vi "test_csm_helper.vi"() -> ()   [LabVIEW 2020]
uses:
  Typedef/Def-Argument Info.ctl
  <userlib>/_NEVSTOP/Communicable State Machine(CSM)/_Support/Priority Queue/Priority Queue.lvclass/Priority Queue.ctl
  <userlib>/_NEVSTOP/Communicable State Machine(CSM)/Utility/Build Error Cluster.vi
  <userlib>/_NEVSTOP/Communicable State Machine(CSM)/_Support/Process/CSMP-Sync Call.vi
  <userlib>/_NEVSTOP/Communicable State Machine(CSM)/Utility/uuid.vi
  <userlib>/_NEVSTOP/Communicable State Machine(CSM)/Utility/Trim Both Whitespace.vi
  <userlib>/_NEVSTOP/Communicable State Machine(CSM)/_Support/Process/CSMP-Async Call.vi
  <userlib>/_NEVSTOP/Communicable State Machine(CSM)/_Support/GlobalEvent/GEvt-Generate Status Log.vi
  <userlib>/_NEVSTOP/Communicable State Machine(CSM)/_Support/Process/CSMP-Broadcast.vi
  <userlib>/_NEVSTOP/Communicable State Machine(CSM)/_Support/GlobalEvent/GEvt-Generate Interrupt Log.vi
  <userlib>/_NEVSTOP/Communicable State Machine(CSM)/_Support/GlobalEvent/GEvt-Generate Register Log.vi
  <userlib>/_NEVSTOP/Communicable State Machine(CSM)/_Support/Process/CSMP-Register Status.vi
  <userlib>/_NEVSTOP/Communicable State Machine(CSM)/_Support/GlobalEvent/GEvt-Generate Unregister Log.vi
  <userlib>/_NEVSTOP/Communicable State Machine(CSM)/_Support/Process/CSMP-Unregister Status.vi
  <userlib>/_NEVSTOP/Communicable State Machine(CSM)/_Support/CSMQ/_CSMObj-Unlock.vi
  <userlib>/_NEVSTOP/Communicable State Machine(CSM)/_Support/Process/CSMP-PostPostMsg.vi
  <userlib>/_NEVSTOP/Communicable State Machine(CSM)/_Support/Process/CSMP-PostSendMsg.vi
  <userlib>/_NEVSTOP/Communicable State Machine(CSM)/_Support/CSMQ/_CSMObj-Lock State.vi
  <userlib>/_NEVSTOP/Communicable State Machine(CSM)/_Support/Common/Splite Reason String Part.vi
  <userlib>/_NEVSTOP/Communicable State Machine(CSM)/_Support/Common/Trim Single line Text.vi
  <userlib>/_NEVSTOP/Communicable State Machine(CSM)/_Support/CSMQ/_CSMOFGV Release.vi
  <userlib>/_NEVSTOP/Communicable State Machine(CSM)/_Support/Common/Remove Comments from Line.vi
  <userlib>/_NEVSTOP/Communicable State Machine(CSM)/_Support/Common/Splite Single-line Message.vi
  <userlib>/_NEVSTOP/Communicable State Machine(CSM)/_Support/Common/Parse Next Single-line State.vi
  <userlib>/_NEVSTOP/Communicable State Machine(CSM)/_Support/CSMQ/_CSMOFGV Dequeue.vi
  <userlib>/_NEVSTOP/Communicable State Machine(CSM)/_Support/CSMQ/_CSMObj-Log Error if in a Remote Session.vi
  <userlib>/_NEVSTOP/Communicable State Machine(CSM)/_Support/GlobalEvent/GEvt-Generate State Change Log.vi
  <userlib>/_NEVSTOP/Communicable State Machine(CSM)/_Support/GlobalEvent/GEvt-Generate Remaining States Log.vi
  <userlib>/_NEVSTOP/Communicable State Machine(CSM)/_Support/GlobalEvent/GEvt-Generate Module Destroyed Log.vi
  <userlib>/_NEVSTOP/Communicable State Machine(CSM)/_Support/GlobalEvent/GEvt-Generate Complete Log.vi
  <userlib>/_NEVSTOP/Communicable State Machine(CSM)/_Support/GlobalEvent/GEvt-Generate Module Created Log.vi
  <userlib>/_NEVSTOP/Communicable State Machine(CSM)/AdvanceAPI/CSM - Revert Arguments-Safe String.vi
  <userlib>/_NEVSTOP/Communicable State Machine(CSM)/AdvanceAPI/CSM - Make String Arguments Safe.vi
  <userlib>/_NEVSTOP/Communicable State Machine(CSM)/_Support/CSMQ/_CSMObj-Message Check.vi
  <userlib>/_NEVSTOP/Communicable State Machine(CSM)/_Support/CSMQ/_CSMObj-Enqueue Cross-Module Message.vi
  <userlib>/_NEVSTOP/Communicable State Machine(CSM)/_Support/CSMQ/_CSMOFGV Get.vi
  <userlib>/_NEVSTOP/Communicable State Machine(CSM)/_Support/FGV-BroadcastRegistry/Cache-Broadcast Registry Search Result.vi
  <userlib>/_NEVSTOP/Communicable State Machine(CSM)/AdvanceAPI/CSM - Register Status Change.vi
  <userlib>/_NEVSTOP/Communicable State Machine(CSM)/AdvanceAPI/CSM - Unregister Status Change.vi
  <userlib>/_NEVSTOP/Communicable State Machine(CSM)/_Support/Common/Hex Str to U8 Data.vi
  <userlib>/_NEVSTOP/Communicable State Machine(CSM)/_Support/Common/Concatenate State with Arguments.vi
  <userlib>/_NEVSTOP/Communicable State Machine(CSM)/_Support/Common/U8 Data to Hex Str.vi
  <userlib>/_NEVSTOP/Communicable State Machine(CSM)/_Support/Priority Queue/Dequeue Element.vi
  <userlib>/_NEVSTOP/Communicable State Machine(CSM)/AdvanceAPI/CSM - Keywords.vi
  <userlib>/_NEVSTOP/Communicable State Machine(CSM)/_Support/Priority Queue/Enqueue Element.vi
  <userlib>/_NEVSTOP/Communicable State Machine(CSM)/_Support/GlobalEvent/FGV-GlobalEventRef.vi
  <userlib>/_NEVSTOP/Communicable State Machine(CSM)/_Support/CSMQ/_CSMOFGV Obtain.vi
  <userlib>/_NEVSTOP/Communicable State Machine(CSM)/_Support/CSMQ/_CSMOFGV.vi
  <userlib>/_NEVSTOP/Communicable State Machine(CSM)/_Support/GlobalEvent/FGV-StatusChangeEventRef.vi
  <userlib>/_NEVSTOP/Communicable State Machine(CSM)/_Support/FGV-BroadcastRegistry/global-CSMQ FGV Change Flag.vi
  <userlib>/_NEVSTOP/Communicable State Machine(CSM)/_Support/FGV-BroadcastRegistry/global-Broadcast Cache Change Flag.vi
  <userlib>/_NEVSTOP/Communicable State Machine(CSM)/_Support/BroadcastRegistry/HelperVI/Broadcast Item Key.vi
  <userlib>/_NEVSTOP/Communicable State Machine(CSM)/_Support/FGV-BroadcastRegistry/FGV-BroadcastRegistry.vi
  <userlib>/_NEVSTOP/Communicable State Machine(CSM)/_Support/Message/Parse Register Message.vi
  <userlib>/_NEVSTOP/Communicable State Machine(CSM)/_Support/Message/Parse Unregister Message.vi
  API/Create From VI Reference.vi
  <userlib>/_NEVSTOP/Communicable State Machine(CSM)/Communicable State Machine.lvlib
  CSM-Helper.lvclass
panel:
  out "Array 3":cluster{string, "Argument":T1, "Response":T1}[](array[cluster])
  out "Array 2":string[](array[string])
  out "Array":string[](array[string])
  out "State History":string
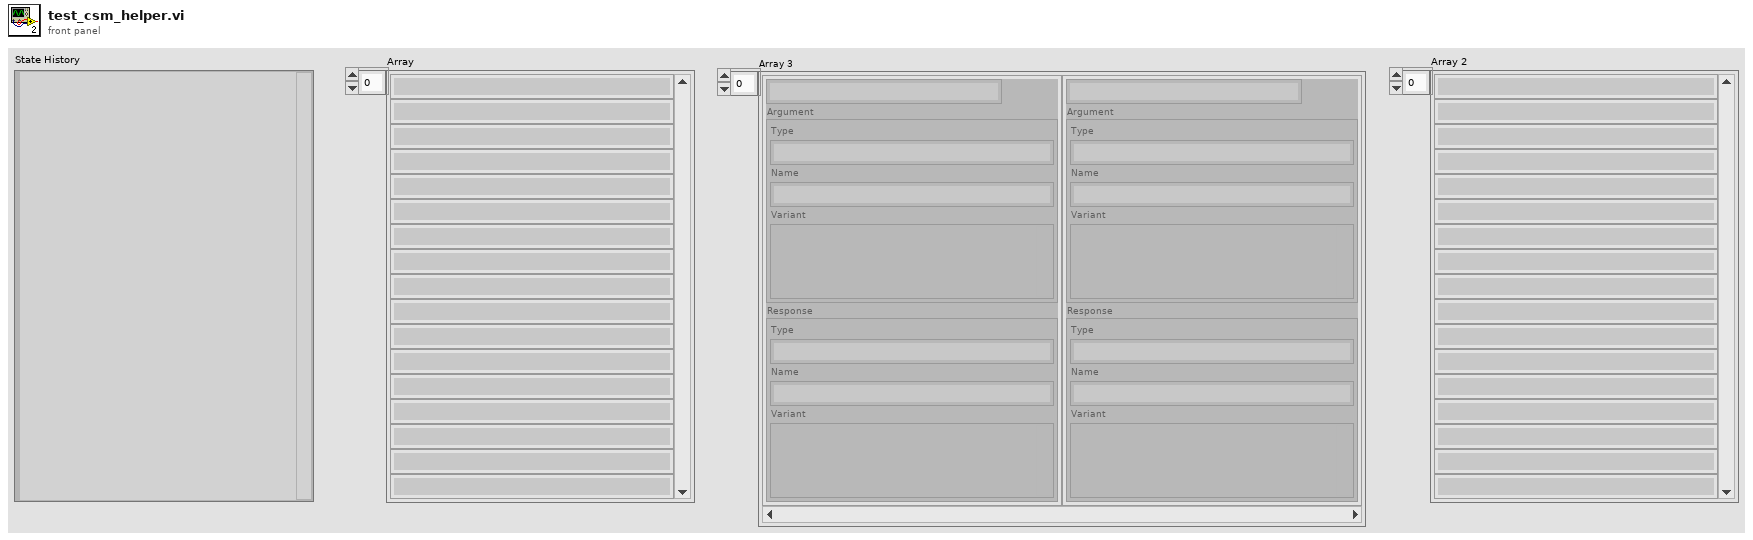
[diagram p1: front panel]
types:
  T1 = typedef "CSM-Helper.lvclass/Def-Argument Info.ctl" = cluster{"Type":string, "Name":string, "Variant":variant}
  T2 = enum32{"Invalid", "Standard", "Closed", "Hidden", "Minimized", "Maximized"}
  T3 = enum32{"invalid app kind", "Development System", "Run Time System", "Student Edition", "Embedded LabVIEW", "Evaluation", "Custom"}
  T4 = typedef "Communicable State Machine.lvlib/_CSM_Response Source Message.ctl" = cluster{"‘State":string, "’Arguments":string, "’Error":errorcluster}
  T5 = cluster{"Core":cluster{"Current VI Reference":refnum<vi>, "Close Panel on Exit?":bool}, "Your Boolean data":bool, "Your string data":string}
  T6 = cluster{"Current VI Reference":refnum<vi>, "Close Panel on Exit?":bool}
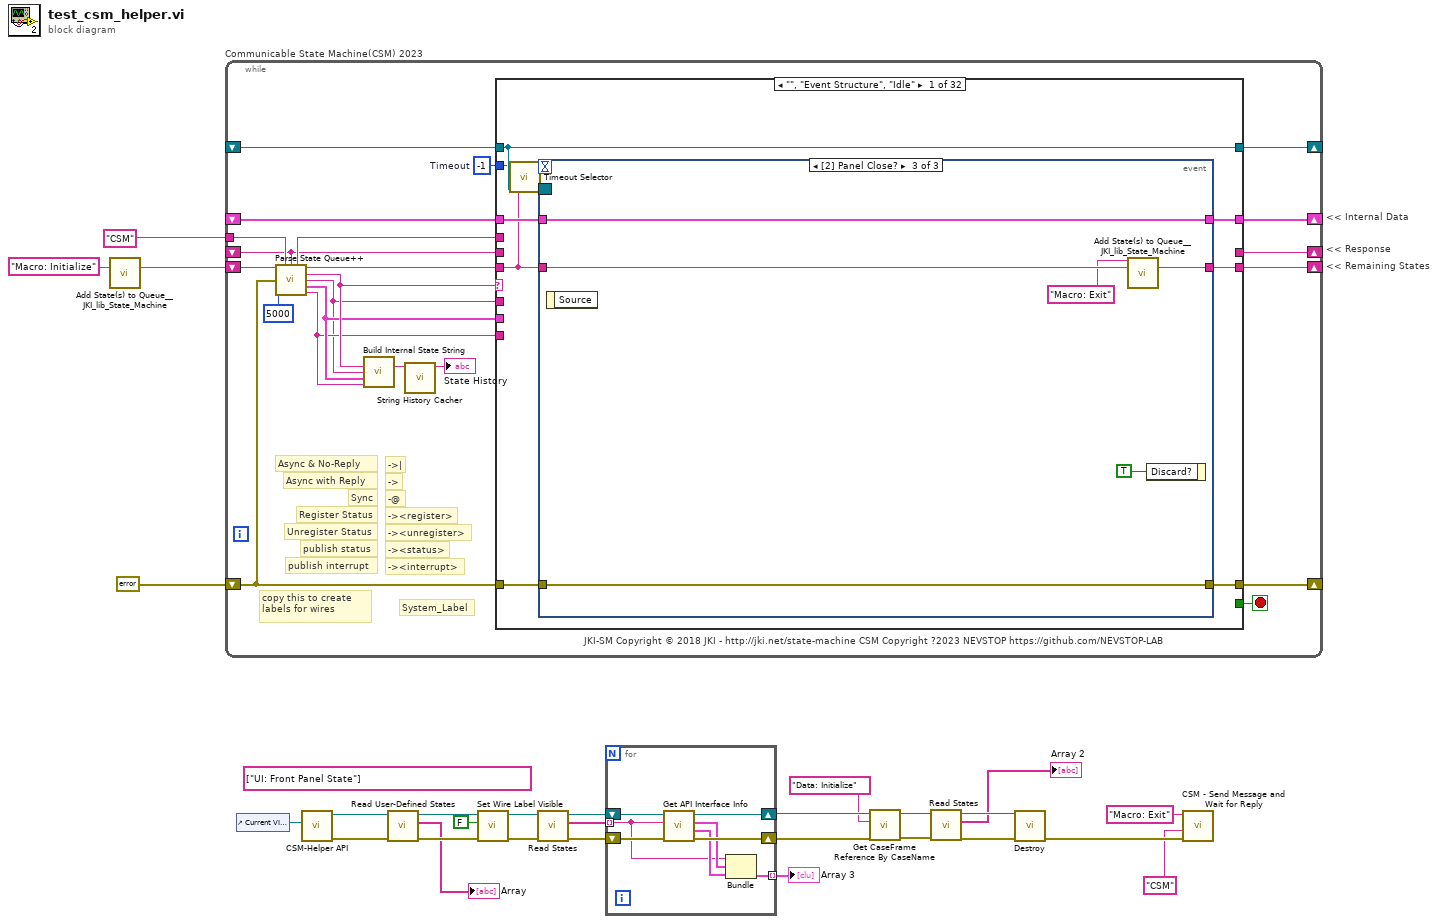
[diagram p0: block diagram]
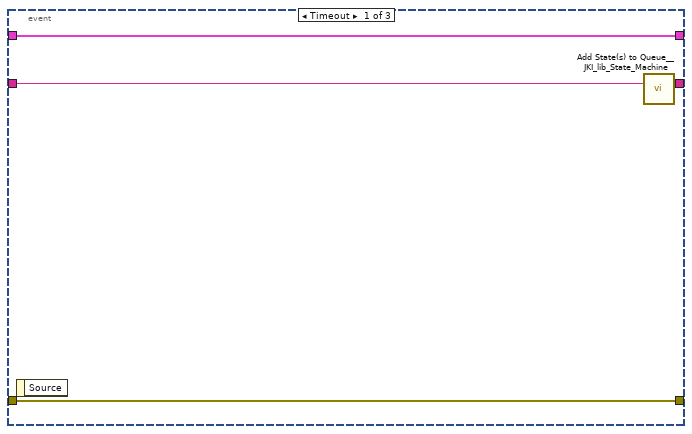
[diagram p2: hidden frame]
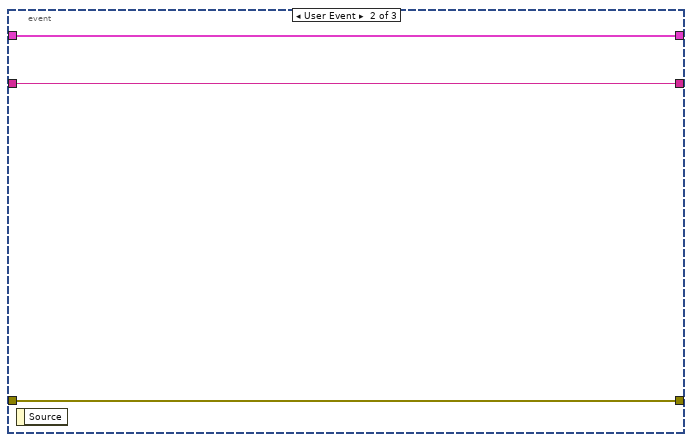
[diagram p3: hidden frame]
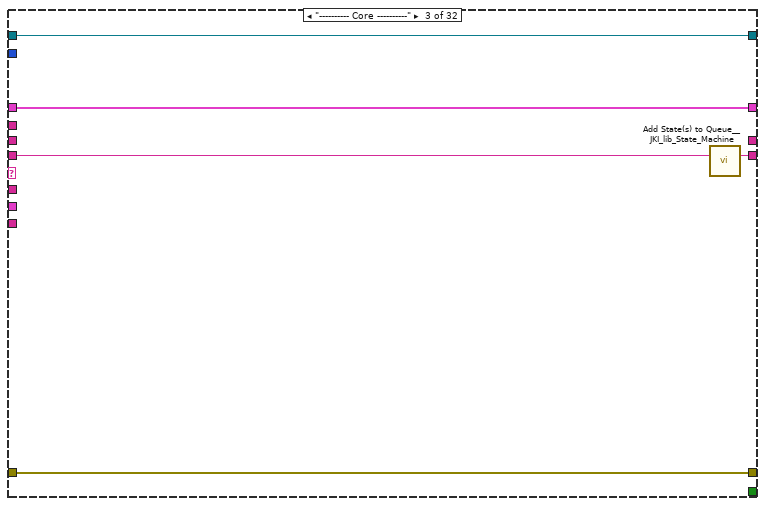
[diagram p5: hidden frame]
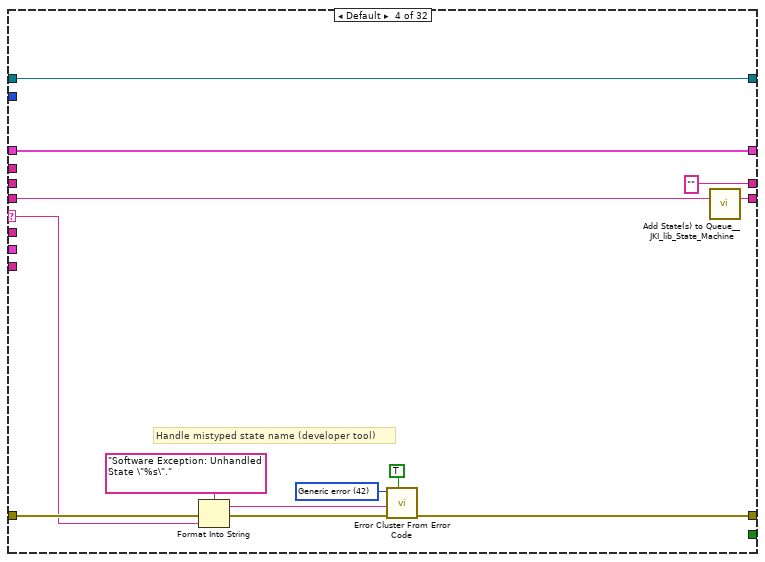
[diagram p6: hidden frame]
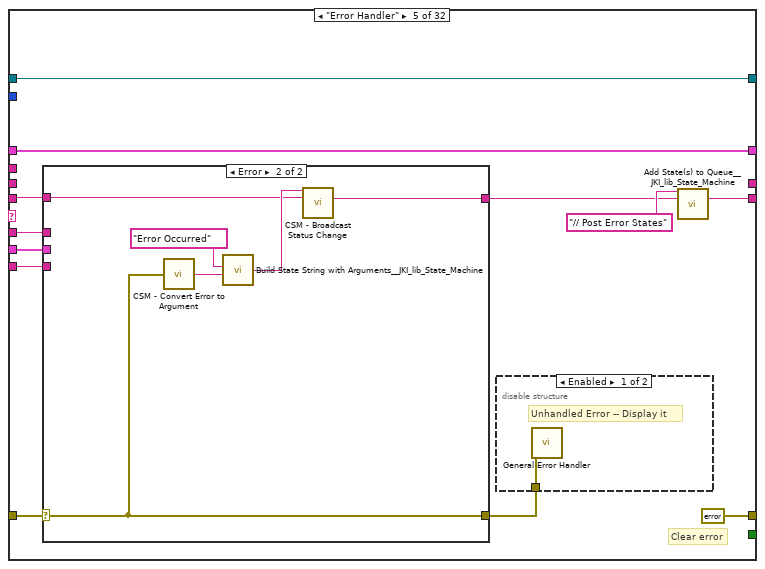
[diagram p7: hidden frame]
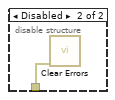
[diagram p8: hidden frame]
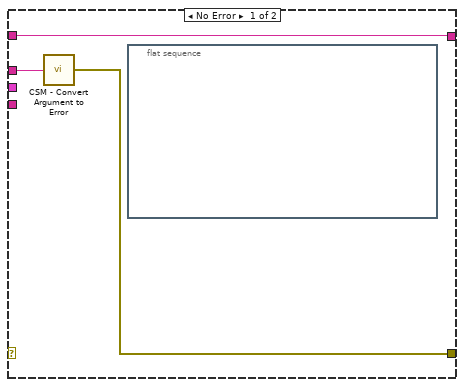
[diagram p9: hidden frame]
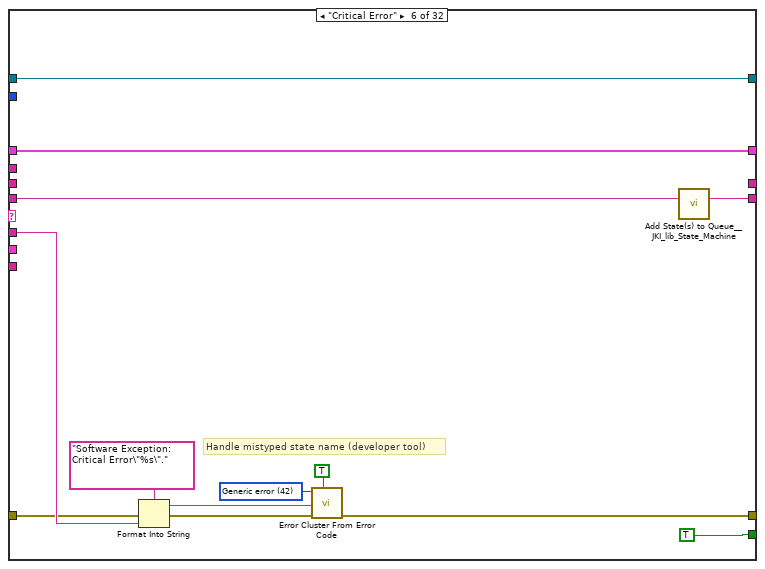
[diagram p10: hidden frame]
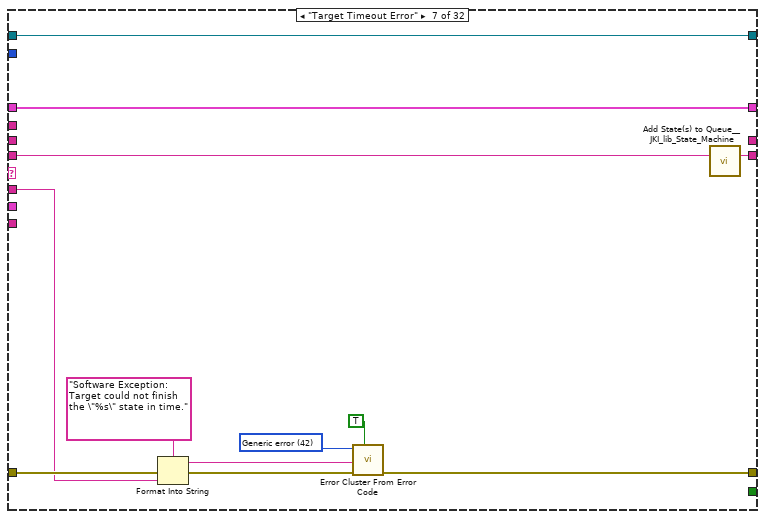
[diagram p11: hidden frame]
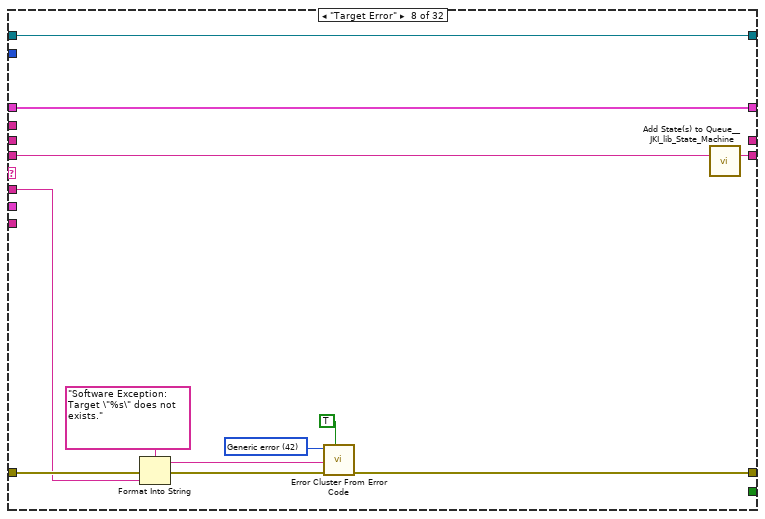
[diagram p12: hidden frame]
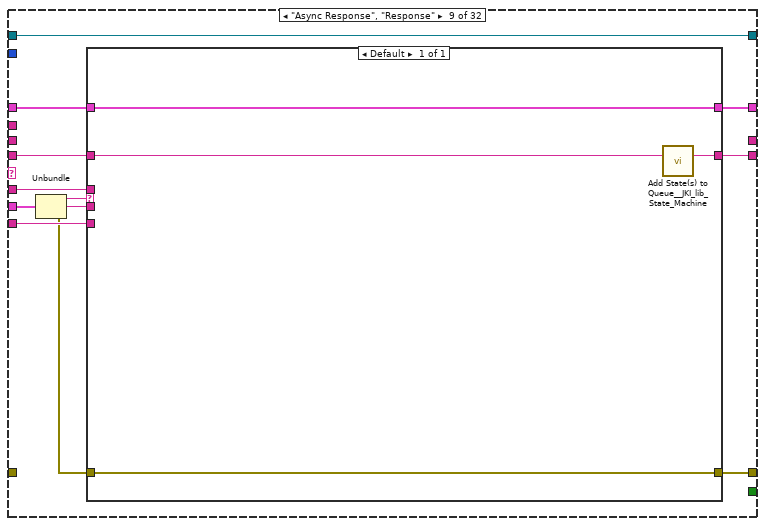
[diagram p13: hidden frame]
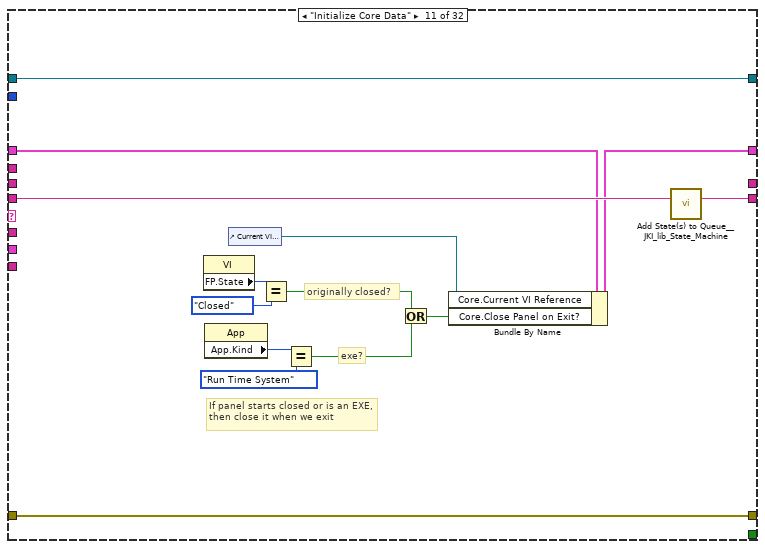
[diagram p15: hidden frame]
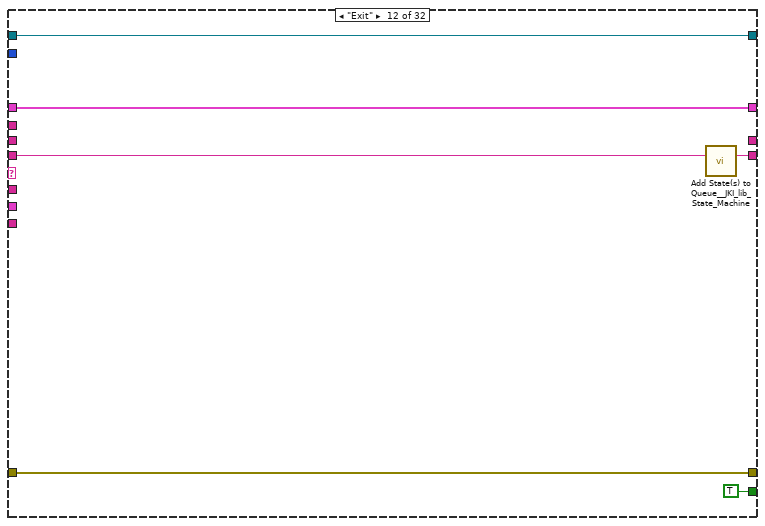
[diagram p16: hidden frame]
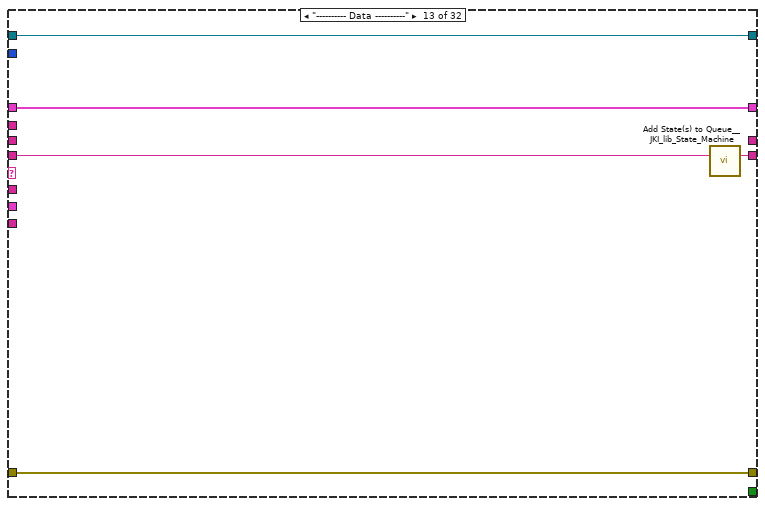
[diagram p17: hidden frame]
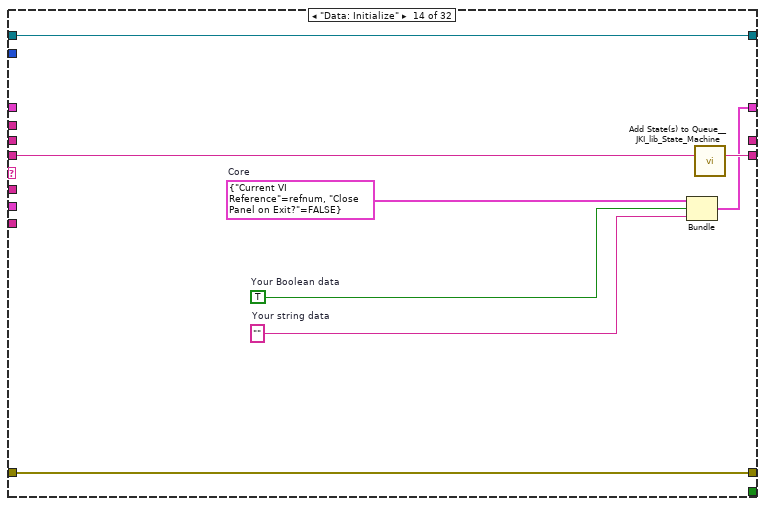
[diagram p18: hidden frame]
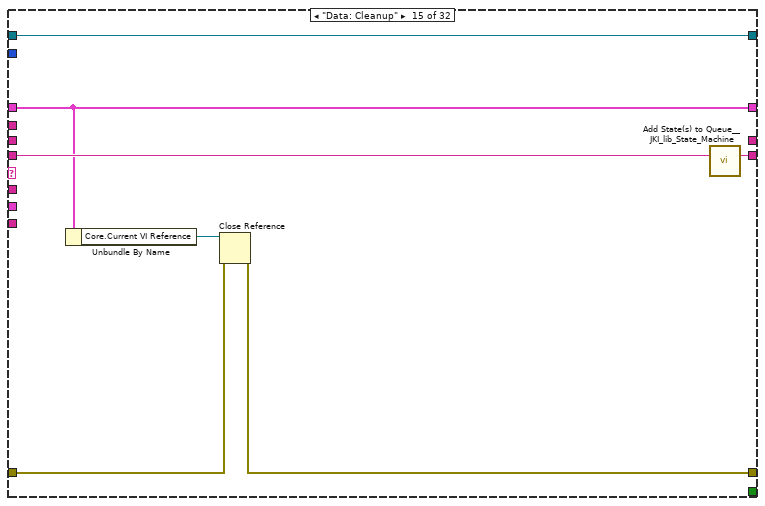
[diagram p19: hidden frame]
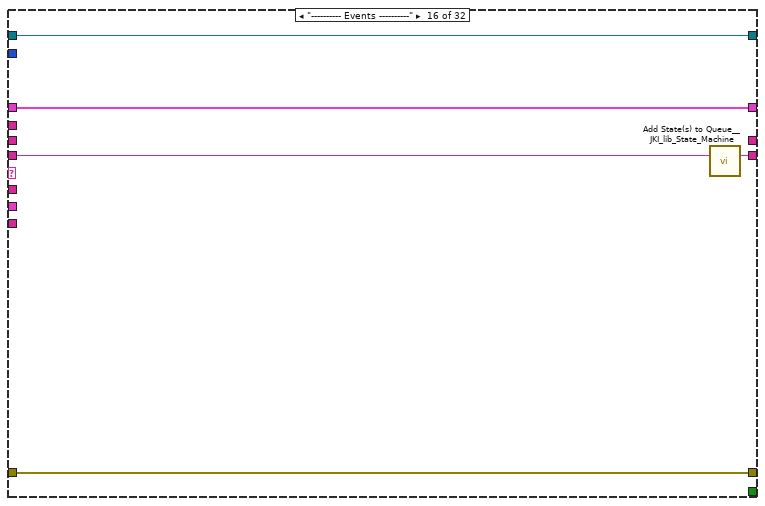
[diagram p20: hidden frame]
diagram:
  (unwired) string[] ["UI: Front Panel State"] ("Array")
  # "<< Internal Data"
  # "<< Response"
  # "<< Remaining States"
  n1 = call <vilib>:"Add State(s) to Queue__JKI_lib_State_Machine.vi"("State(s) in (\"\")"="Macro: Initialize" ("Init State(\"Macro: Initialize\")")) -> ("States Out"=w25:string)  [unwired: 14 in]
  n2 = while "Communicable State Machine(CSM) 2023" {
    shift-right: [w45] -> _
    shift-left: _ -> [w44]
    shift-right: [w48] -> _
    shift-left: errorcluster {"status"=FALSE, "code"=0, "source"=""} ("error out") -> [w42]
    shift-right: [w47] -> _
    shift-left: w25 -> [w49]
    tunnel: "CSM" ("Name(\"\" to use uuid)") -> [w37]
    shift-right: [w40] -> _
    shift-left: _ -> [w30]
    shift-right: [w39] -> _
    shift-left: _ -> [w38]
    stop <- w46 stop-if-true
    w43 = -1  # Timeout
    # "-><interrupt>"
    # "-><status>"
    # "-><unregister>"
    # "-><register>"
    # "-@"
    # "->"
    # "->|"
    # "publish interrupt"
    # "publish status"
    # "Unregister Status"
    # "Register Status"
    # "Sync"
    # "Async with Reply"
    # "Async & No-Reply"
    # "copy this to create labels for wires"
    # "System_Label"
    # "JKI-SM Copyright © 2018 JKI - http://jki.net/state-machine CSM Copyright ?2023 NEVSTOP https://github.com/NEVSTOP-LAB"
    n3 = call <userlib>:"Parse State Queue++.vi"("State Queue"=w49, "Name(\"\" to use uuid)"=w37, "Response Arguments"=w30, "Error In (no error)"=w42, "Response Timeout(5000ms)"=5000 ("Response Timeout(1000ms)")) -> ("Name Used"=w31:string, "Remaining States"=w50:string, "Current State"=w34:string, "Arguments"=w29:string, ">> Response Source Message >>"=w33:T4, ">> Source CSM >>"=w32:string)  [unwired: 5 in]
    n4 = call <userlib>:"Build Internal State String.vi"("State"=w34, "Arguments (\"\")"=w29, ">> Response Source Message >>"=w33, "Source (\"\")"=w32) -> ("State with Arguments"=w35:string)  [unwired: 11 in]
    n5 = call <userlib>:"String History Cacher.vi"("String"=w35) -> ("String Cache"=→"State History":string)  [unwired: 10 in]
    n6 = case shown="\"\", \"Event Structure\", \"Idle\"" w34 {
      selector: w34 -> [_ _ _ w84 _ _ _ _ _ _ _ _ _ _ _ _ _ _ _ _ _ _ _ _ _ _ _ _ _ _ _ _]
      tunnel: w50 -> [w51 w76 w81 w88 w99 w129 w137 w149 w164 w173 w188 w194 w199 w207 w214 w219 w226 w230 w236 w241 w248 w264 w334 w340 w352 w355 w361 w365 w369 w376 w381 w386]
      tunnel: w29 -> [_ _ _ _ w97 w122 w133 w145 w158 _ _ _ _ _ _ _ _ _ _ _ w243 w258 _ _ _ _ w357 _ _ _ _ _]
      tunnel: w44 -> [w58 w75 w78 w86 w105 w130 w135 w147 w162 w172 w181 w192 w196 _ w209 w216 w225 w229 w233 w239 w246 w260 w331 w337 w349 w354 w360 w364 w368 w373 w378 w383]
      tunnel: [w57 w74 w79 w90 errorcluster {"status"=FALSE, "code"=0, "source"=""} ("error out") w118 w131 w143 w161 w174 w185 w191 w197 w204 w210 w217 w220 w228 w234 w238 w244 w261 w332 w338 w350 w356 w362 w366 w370 w374 w379 w384] -> w48
      tunnel: w42 -> [w56 w74 w79 w89 w103 w119 w138 w150 _ w174 w185 w191 w197 w204 w211 w217 _ w231 w234 w238 w245 w262 w332 w338 w350 w356 w362 w366 w370 w374 w379 w384]
      tunnel: [w59 w76 w80 w87 w101 w128 w136 w148 w165 w173 w187 w193 w198 w206 w213 w218 w226 w230 w235 w240 w247 w263 w333 w339 w351 w355 w361 w365 w369 w375 w380 w385] -> w47
      tunnel: [_ _ _ _ _ TRUE _ _ _ _ _ TRUE _ _ _ _ _ _ _ _ _ _ _ _ _ _ _ _ _ _ _ _] -> w46
      tunnel: [w55 w75 w78 w86 w105 w130 w135 w147 w163 w172 w186 w192 w196 w205 w209 w216 w225 w229 w233 w239 w246 w260 w331 w337 w349 w354 w360 w364 w368 w373 w378 w383] -> w45
      tunnel: w43 -> [w53 _ _ _ _ _ _ _ _ _ _ _ _ _ _ _ _ _ _ _ _ _ _ _ _ _ _ _ _ _ _ _]
      tunnel: w32 -> [_ _ _ _ w96 _ _ _ w159 _ _ _ _ _ _ _ _ _ _ _ _ _ _ _ _ _ _ _ _ _ _ _]
      tunnel: w33 -> [_ _ _ _ w95 _ _ _ w160 _ _ _ _ _ _ _ _ _ _ _ _ _ _ _ _ _ _ _ _ _ _ _]
      tunnel: [_ _ _ "" _ _ _ _ _ _ _ _ _ _ _ _ _ _ _ _ _ _ _ _ _ _ "API1 Response" _ _ _ _ _] -> w40
      tunnel: [w54 w73 w77 w82 w104 w120 w132 w144 w166 w171 w175 w189 w195 w200 w208 w215 w224 w227 w232 w237 w242 w257 w330 w335 w342 w353 w359 w363 w367 w372 w377 w382] -> w39
      tunnel: w38 -> [w54 w73 w77 w82 w104 w120 w132 w144 w166 w171 w175 w189 w195 w200 w208 w215 _ w227 w232 w237 w242 w257 w330 w335 w342 w353 w359 w363 w367 w372 w377 w382]
      tunnel: w31 -> [_ _ _ _ _ _ _ _ _ _ _ _ _ _ _ _ w223 _ _ _ _ _ _ _ _ _ _ _ _ _ _ _]
      tunnel: w30 -> [_ _ _ _ _ _ _ _ _ _ _ _ _ _ _ _ _ _ _ _ _ _ _ _ _ _ _ _ _ _ _ _]
      frame "", "Event Structure", "Idle" {
        n7 = call <userlib>:"Timeout Selector.vi"("Remaining States"=w51, "Timeout Expected"=w53) -> ("Timeout"=w52:i32)  [unwired: 5 in]
        n8 = event shown="[2] Panel Close?" {
          selector: w54 -> [_ _ _]
          dyn-events: _ -> [_ _ _]
          timeout: w52 -> [_ _ _]
          tunnel: w51 -> [w63 w65 w72]
          tunnel: [w62 w65 w71] -> w59
          tunnel: w58 -> [w60 w66 w69]
          tunnel: [w61 w64 w70] -> w57
          tunnel: w56 -> [w61 w64 w70]
          tunnel: [w60 w66 w69] -> w55
          event Timeout {
            n9 = event-data() -> ()  [unwired: 1 in, 1 out]
            n10 = call <vilib>:"Add State(s) to Queue__JKI_lib_State_Machine.vi"("State(s) in (\"\")"=w63) -> ("States Out"=w62:string)  [unwired: 14 in]
          }
          event User Event {
            n11 = event-data() -> ()  [unwired: 1 in, 1 out]
          }
          event Panel Close? {
            n12 = event-data() -> ()  [unwired: 1 in, 1 out]
            n13 = call <vilib>:"Add State(s) to Queue__JKI_lib_State_Machine.vi"("State(s) in Front (\"\")"="Macro: Exit", "State(s) in (\"\")"=w72) -> ("States Out"=w71:string)  [unwired: 13 in]
            n14 = event-data("Discard?"=TRUE) -> ()  [unwired: 1 in, 1 out]
          }
        }
      }
      frame "CSM Documentation" {
      }
      frame "---------- Core ----------" {
        n15 = call <vilib>:"Add State(s) to Queue__JKI_lib_State_Machine.vi"("State(s) in (\"\")"=w81) -> ("States Out"=w80:string)  [unwired: 14 in]
      }
      frame Default {
        w93 = 42 items=["No error", "Argument error", "Memory is full", "Out of zone", "End of file", "File already open", "Generic file I/O error", "File not found", "File permission error", "Disk is full", "Duplicate path", "Too many files open", "System feature not enabled", "Resource file not found", "Cannot add resource", "Resource not found", "Image not found", "Image memory error", "Pen does not exist", "Config type invalid", "Config token not found", "Config parse error", "Config memory error", "Bad external code format", "Bad external code offset", "External code not present", "Null window", "Destroy window error", "Null menu", "Print aborted", "Bad print record", "Print driver error", "Windows error during printing", "Memory error during printing", "Print dialog error", "Generic print error", "Invalid device refnum", "Device not found", "Device parameter error", "Device unit error", "Cannot open device", "Device call aborted", "Generic error", "Cancelled by user", "Object ID too low", "Object ID too high", "Object not in heap", "Unknown heap", "Unknown object (invalid DefProc)", "Unknown object (DefProc not in table)", "Message out of range", "Invalid (null) method", "Unknown message", "Manager call not supported", "Bad address", "Network operation in progress", "Network operation timed out", "Connection is busy", "Network attribute not supported", "Network error", "Address in use", "System out of memory", "Connection aborted", "Connection refused", "Not connected", "Already connected", "Connection closed", "Initialization error (interapplication manager)", "Bad occurrence", "Wait on unbound occurrence handler", "Occurrence queue overflow", "Datalog type conflict", "Unused", "Unrecognized type (interapplication manager)", "Memory corrupt", "Failed to make temporary DLL", "Old CIN version", "Drag socket not found", "Failed to load drop-object", "Failed to register OLE object", "Failed to release OLE object", "Format specifier type mismatch", "Unknown format specifier", "Too few format specifiers", "Too many format specifiers", "Scan failed", "Newer CIN version", "Error converting to variant", "Runtime menu error", "Password tampered", "Variant attribute not found", "Incompatible variant data type", "Event data is not available", "Event Store is not present", "Occurrence is not found", "Event Queue is not created", "Event info is not available", "Refnum passed is NULL", "Error retrieving Class GUID", "Error retrieving CoClass GUID", "Error retrieving TypeLib GUID.", "Bad built application magic bytes.", "Specific driver is different from the specific driver associated with the Logical Name.", "There is no session opened to the class driver.", "Max Error", "MAX - Error with config objects", "MAX - Error loading configuration", "MAX - Group not supported"]
        # "Handle mistyped state name (developer tool)"
        n16 = Format Into String(format string="Software Exception: Unhandled State \"%s\"." ("message"), error in=w89, w84) -> (resulting string=w92:string, error out=w91:errorcluster)  [unwired: 1 in]
        n17 = call <vilib>:"Error Cluster From Error Code.vi"("show call chain? (False)"=TRUE, "error in (no error)"=w91, "error message (\"\")"=w92, "error code (0)"=w93) -> ("error out"=w90:errorcluster)  [unwired: 5 in]
        n18 = call <vilib>:"Add State(s) to Queue__JKI_lib_State_Machine.vi"("State(s) in (\"\")"=w88) -> ("States Out"=w87:string)  [unwired: 14 in]
      }
      frame "Error Handler" {
        # "Clear error"
        n19 = case shown="Error" w103 {
          selector: w103 -> [_ w112]
          tunnel: [w110 w114] -> w100
          tunnel: w99 -> [w110 w113]
          tunnel: [w109 w112] -> w98
          tunnel: w97 -> [w111 _]
          tunnel: w96 -> [_ _]
          tunnel: w95 -> [_ _]
          frame No Error {
            n20 = call <userlib>:"CSM - Convert Argument to Error.vi"("Argument"=w111) -> ("error"=w109:errorcluster)  [unwired: 4 in]
            n21 = flat-sequence {
              frame #0 {
              }
            }
          }
          frame Error {
            n22 = call <userlib>:"CSM - Convert Error to Argument.vi"("error in (no error)"=w112) -> ("Arguments"=w116:string)  [unwired: 4 in]
            n23 = call <vilib>:"Build State String with Arguments__JKI_lib_State_Machine.vi"("Arguments (\"\")"=w116, "State"="Error Occurred" ("Status with Arguments")) -> ("State with Arguments"=w115:string)  [unwired: 4 in]
            n24 = call <userlib>:"CSM - Broadcast Status Change.vi"("Status with Arguments"=w115, "State Queue"=w113) -> ("Remaining States"=w114:string)  [unwired: 13 in]
          }
        }
        n25 = disable-structure shown="Enabled" {
          disable-tunnel: w98 -> [w107 w108]
          frame Enabled {
            # "Unhandled Error -- Display it"
            n26 = call <vilib>:"General Error Handler.vi"("error in (no error)"=w107) -> ()  [unwired: 10 in, 5 out]
          }
          frame Disabled {
            n27 = call <vilib>:"Clear Errors.vi"("error in (no error)"=w108) -> ()  [unwired: 5 in, 2 out]
          }
        }
        n28 = call <vilib>:"Add State(s) to Queue__JKI_lib_State_Machine.vi"("State(s) in Front (\"\")"="// Post Error States", "State(s) in (\"\")"=w100) -> ("States Out"=w101:string)  [unwired: 13 in]
      }
      frame "Critical Error" {
        w126 = 42 items=["No error", "Argument error", "Memory is full", "Out of zone", "End of file", "File already open", "Generic file I/O error", "File not found", "File permission error", "Disk is full", "Duplicate path", "Too many files open", "System feature not enabled", "Resource file not found", "Cannot add resource", "Resource not found", "Image not found", "Image memory error", "Pen does not exist", "Config type invalid", "Config token not found", "Config parse error", "Config memory error", "Bad external code format", "Bad external code offset", "External code not present", "Null window", "Destroy window error", "Null menu", "Print aborted", "Bad print record", "Print driver error", "Windows error during printing", "Memory error during printing", "Print dialog error", "Generic print error", "Invalid device refnum", "Device not found", "Device parameter error", "Device unit error", "Cannot open device", "Device call aborted", "Generic error", "Cancelled by user", "Object ID too low", "Object ID too high", "Object not in heap", "Unknown heap", "Unknown object (invalid DefProc)", "Unknown object (DefProc not in table)", "Message out of range", "Invalid (null) method", "Unknown message", "Manager call not supported", "Bad address", "Network operation in progress", "Network operation timed out", "Connection is busy", "Network attribute not supported", "Network error", "Address in use", "System out of memory", "Connection aborted", "Connection refused", "Not connected", "Already connected", "Connection closed", "Initialization error (interapplication manager)", "Bad occurrence", "Wait on unbound occurrence handler", "Occurrence queue overflow", "Datalog type conflict", "Unused", "Unrecognized type (interapplication manager)", "Memory corrupt", "Failed to make temporary DLL", "Old CIN version", "Drag socket not found", "Failed to load drop-object", "Failed to register OLE object", "Failed to release OLE object", "Format specifier type mismatch", "Unknown format specifier", "Too few format specifiers", "Too many format specifiers", "Scan failed", "Newer CIN version", "Error converting to variant", "Runtime menu error", "Password tampered", "Variant attribute not found", "Incompatible variant data type", "Event data is not available", "Event Store is not present", "Occurrence is not found", "Event Queue is not created", "Event info is not available", "Refnum passed is NULL", "Error retrieving Class GUID", "Error retrieving CoClass GUID", "Error retrieving TypeLib GUID.", "Bad built application magic bytes.", "Specific driver is different from the specific driver associated with the Logical Name.", "There is no session opened to the class driver.", "Max Error", "MAX - Error with config objects", "MAX - Error loading configuration", "MAX - Group not supported"]
        # "Handle mistyped state name (developer tool)"
        n29 = Format Into String(format string="Software Exception: Critical Error\"%s\"." ("message"), error in=w119, w122) -> (resulting string=w125:string, error out=w124:errorcluster)  [unwired: 1 in]
        n30 = call <vilib>:"Error Cluster From Error Code.vi"("show call chain? (False)"=TRUE, "error in (no error)"=w124, "error message (\"\")"=w125, "error code (0)"=w126) -> ("error out"=w118:errorcluster)  [unwired: 5 in]
        n31 = call <vilib>:"Add State(s) to Queue__JKI_lib_State_Machine.vi"("State(s) in (\"\")"=w129) -> ("States Out"=w128:string)  [unwired: 14 in]
      }
      frame "Target Timeout Error" {
        w141 = 42 items=["No error", "Argument error", "Memory is full", "Out of zone", "End of file", "File already open", "Generic file I/O error", "File not found", "File permission error", "Disk is full", "Duplicate path", "Too many files open", "System feature not enabled", "Resource file not found", "Cannot add resource", "Resource not found", "Image not found", "Image memory error", "Pen does not exist", "Config type invalid", "Config token not found", "Config parse error", "Config memory error", "Bad external code format", "Bad external code offset", "External code not present", "Null window", "Destroy window error", "Null menu", "Print aborted", "Bad print record", "Print driver error", "Windows error during printing", "Memory error during printing", "Print dialog error", "Generic print error", "Invalid device refnum", "Device not found", "Device parameter error", "Device unit error", "Cannot open device", "Device call aborted", "Generic error", "Cancelled by user", "Object ID too low", "Object ID too high", "Object not in heap", "Unknown heap", "Unknown object (invalid DefProc)", "Unknown object (DefProc not in table)", "Message out of range", "Invalid (null) method", "Unknown message", "Manager call not supported", "Bad address", "Network operation in progress", "Network operation timed out", "Connection is busy", "Network attribute not supported", "Network error", "Address in use", "System out of memory", "Connection aborted", "Connection refused", "Not connected", "Already connected", "Connection closed", "Initialization error (interapplication manager)", "Bad occurrence", "Wait on unbound occurrence handler", "Occurrence queue overflow", "Datalog type conflict", "Unused", "Unrecognized type (interapplication manager)", "Memory corrupt", "Failed to make temporary DLL", "Old CIN version", "Drag socket not found", "Failed to load drop-object", "Failed to register OLE object", "Failed to release OLE object", "Format specifier type mismatch", "Unknown format specifier", "Too few format specifiers", "Too many format specifiers", "Scan failed", "Newer CIN version", "Error converting to variant", "Runtime menu error", "Password tampered", "Variant attribute not found", "Incompatible variant data type", "Event data is not available", "Event Store is not present", "Occurrence is not found", "Event Queue is not created", "Event info is not available", "Refnum passed is NULL", "Error retrieving Class GUID", "Error retrieving CoClass GUID", "Error retrieving TypeLib GUID.", "Bad built application magic bytes.", "Specific driver is different from the specific driver associated with the Logical Name.", "There is no session opened to the class driver.", "Max Error", "MAX - Error with config objects", "MAX - Error loading configuration", "MAX - Group not supported"]
        n32 = Format Into String(format string="Software Exception: Target could not finish the \"%s\" state in time." ("message"), error in=w138, w133) -> (resulting string=w140:string, error out=w139:errorcluster)  [unwired: 1 in]
        n33 = call <vilib>:"Error Cluster From Error Code.vi"("show call chain? (False)"=TRUE, "error in (no error)"=w139, "error message (\"\")"=w140, "error code (0)"=w141) -> ("error out"=w131:errorcluster)  [unwired: 5 in]
        n34 = call <vilib>:"Add State(s) to Queue__JKI_lib_State_Machine.vi"("State(s) in (\"\")"=w137) -> ("States Out"=w136:string)  [unwired: 14 in]
      }
      frame "Target Error" {
        w153 = 42 items=["No error", "Argument error", "Memory is full", "Out of zone", "End of file", "File already open", "Generic file I/O error", "File not found", "File permission error", "Disk is full", "Duplicate path", "Too many files open", "System feature not enabled", "Resource file not found", "Cannot add resource", "Resource not found", "Image not found", "Image memory error", "Pen does not exist", "Config type invalid", "Config token not found", "Config parse error", "Config memory error", "Bad external code format", "Bad external code offset", "External code not present", "Null window", "Destroy window error", "Null menu", "Print aborted", "Bad print record", "Print driver error", "Windows error during printing", "Memory error during printing", "Print dialog error", "Generic print error", "Invalid device refnum", "Device not found", "Device parameter error", "Device unit error", "Cannot open device", "Device call aborted", "Generic error", "Cancelled by user", "Object ID too low", "Object ID too high", "Object not in heap", "Unknown heap", "Unknown object (invalid DefProc)", "Unknown object (DefProc not in table)", "Message out of range", "Invalid (null) method", "Unknown message", "Manager call not supported", "Bad address", "Network operation in progress", "Network operation timed out", "Connection is busy", "Network attribute not supported", "Network error", "Address in use", "System out of memory", "Connection aborted", "Connection refused", "Not connected", "Already connected", "Connection closed", "Initialization error (interapplication manager)", "Bad occurrence", "Wait on unbound occurrence handler", "Occurrence queue overflow", "Datalog type conflict", "Unused", "Unrecognized type (interapplication manager)", "Memory corrupt", "Failed to make temporary DLL", "Old CIN version", "Drag socket not found", "Failed to load drop-object", "Failed to register OLE object", "Failed to release OLE object", "Format specifier type mismatch", "Unknown format specifier", "Too few format specifiers", "Too many format specifiers", "Scan failed", "Newer CIN version", "Error converting to variant", "Runtime menu error", "Password tampered", "Variant attribute not found", "Incompatible variant data type", "Event data is not available", "Event Store is not present", "Occurrence is not found", "Event Queue is not created", "Event info is not available", "Refnum passed is NULL", "Error retrieving Class GUID", "Error retrieving CoClass GUID", "Error retrieving TypeLib GUID.", "Bad built application magic bytes.", "Specific driver is different from the specific driver associated with the Logical Name.", "There is no session opened to the class driver.", "Max Error", "MAX - Error with config objects", "MAX - Error loading configuration", "MAX - Group not supported"]
        n35 = Format Into String(format string="Software Exception: Target \"%s\" does not exists." ("message"), error in=w150, w145) -> (resulting string=w152:string, error out=w151:errorcluster)  [unwired: 1 in]
        n36 = call <vilib>:"Error Cluster From Error Code.vi"("show call chain? (False)"=TRUE, "error in (no error)"=w151, "error message (\"\")"=w152, "error code (0)"=w153) -> ("error out"=w143:errorcluster)  [unwired: 5 in]
        n37 = call <vilib>:"Add State(s) to Queue__JKI_lib_State_Machine.vi"("State(s) in (\"\")"=w149) -> ("States Out"=w148:string)  [unwired: 14 in]
      }
      frame "Async Response", "Response" {
        n38 = Unbundle(w160) -> ("‘State"=w157:string, "’Arguments"=w156:string, "’Error"=w155:errorcluster)
        n39 = case shown="Default" w157 {
          tunnel: [w167] -> w165
          tunnel: w164 -> [w168]
          tunnel: [w170] -> w163
          tunnel: w162 -> [w170]
          tunnel: [w169] -> w161
          tunnel: w155 -> [w169]
          tunnel: w159 -> [_]
          tunnel: w158 -> [_]
          tunnel: w156 -> [_]
          frame Default {
            n40 = call <vilib>:"Add State(s) to Queue__JKI_lib_State_Machine.vi"("State(s) in (\"\")"=w168) -> ("States Out"=w167:string)  [unwired: 14 in]
          }
        }
      }
      frame "Async Message Posted" {
      }
      frame "Initialize Core Data" {
        # "originally closed?"
        # "exe?"
        # "If panel starts closed or is an EXE, then close it when we exit"
        n41 = property class="VI"() -> ("FP.State"=w178:T2)  [unwired: 2 in, 2 out]
        n42 = property class="App"() -> ("App.Kind"=w184:T3)  [unwired: 2 in, 2 out]
        n43 = control-ref of="Current VI Reference"() -> (w179:refnum<vi>)
        n44 = Equal?(x=w178, y=T2."Closed" ("Front Panel Window:State")) -> (x = y?=w176:bool)
        n45 = Equal?(x=w184, y=T3."Run Time System" ("Application:Kind")) -> (x = y?=w182:bool)
        n46 = Or(x=w176, y=w182) -> (x .or. y?=w180:bool)
        n47 = Bundle By Name(cluster=w181, "Core.Current VI Reference"=w179, "Core.Close Panel on Exit?"=w180) -> (w186:T5)
        n48 = call <vilib>:"Add State(s) to Queue__JKI_lib_State_Machine.vi"("State(s) in (\"\")"=w188) -> ("States Out"=w187:string)  [unwired: 14 in]
      }
      frame "Exit" {
        n49 = call <vilib>:"Add State(s) to Queue__JKI_lib_State_Machine.vi"("State(s) in (\"\")"=w194) -> ("States Out"=w193:string)  [unwired: 14 in]
      }
      frame "---------- Data ----------" {
        n50 = call <vilib>:"Add State(s) to Queue__JKI_lib_State_Machine.vi"("State(s) in (\"\")"=w199) -> ("States Out"=w198:string)  [unwired: 14 in]
      }
      frame "Data: Initialize" {
        w201 = T6 {"Current VI Reference"=refnum, "Close Panel on Exit?"=FALSE}  # Core
        w203 = TRUE  # Your Boolean data
        w202 = ""  # Your string data
        n51 = Bundle("Core"=w201, "Your Boolean data"=w203, "Your string data"=w202) -> (w205:T5)  [unwired: 1 in]
        n52 = call <vilib>:"Add State(s) to Queue__JKI_lib_State_Machine.vi"("State(s) in (\"\")"=w207) -> ("States Out"=w206:string)  [unwired: 14 in]
      }
      frame "Data: Cleanup" {
        n53 = Unbundle By Name(w209) -> ("Core.Current VI Reference"=w212:refnum<vi>)
        n54 = Close Reference(reference=w212, error in (no error)=w211) -> (error out=w210:errorcluster)
        n55 = call <vilib>:"Add State(s) to Queue__JKI_lib_State_Machine.vi"("State(s) in (\"\")"=w214) -> ("States Out"=w213:string)  [unwired: 14 in]
      }
      frame "---------- Events ----------" {
        n56 = call <vilib>:"Add State(s) to Queue__JKI_lib_State_Machine.vi"("State(s) in (\"\")"=w219) -> ("States Out"=w218:string)  [unwired: 14 in]
      }
      frame "Events: Register" {
        n57 = call <userlib>:"CSM - Get New State Notifier Event.vi"("Name(\"\" to use uuid) in"=w223) -> ("Error out"=w221:errorcluster, "New State Notifier Event"=w222:refnum<user-event>)  [unwired: 9 in]
        n58 = register-events(error in=w221, w222) -> (reference out=w224:refnum<event-registration>, error out=w220:errorcluster)  [unwired: 1 in]
      }
      frame "Events: Unregister" {
        n59 = Unregister For Events(event registration refnum=w227, error in=w231) -> (error out=w228:errorcluster)
      }
      frame "---------- UI ----------" {
        n60 = call <vilib>:"Add State(s) to Queue__JKI_lib_State_Machine.vi"("State(s) in (\"\")"=w236) -> ("States Out"=w235:string)  [unwired: 14 in]
      }
      frame "UI: Initialize" {
        n61 = call <vilib>:"Add State(s) to Queue__JKI_lib_State_Machine.vi"("State(s) in (\"\")"=w241) -> ("States Out"=w240:string)  [unwired: 14 in]
      }
      frame "UI: Cursor Set" {
        # "Argument"
        n62 = disable-structure "Conditional Disable Structure" shown="Default" {
          disable-tunnel: w245 -> [w251 w256]
          disable-tunnel: [w250 w256] -> w244
          disable-tunnel: w243 -> [w249 _]
          frame condition #0 (active) {
            n63 = case shown="\"Busy\"" w249 {
              tunnel: w251 -> [w253 w255]
              tunnel: [w252 w254] -> w250
              frame "Idle", Default {
                n64 = call <vilib>:"Unset Busy.vi"("error in (no error)"=w253) -> ("error out"=w252:errorcluster)  [unwired: 10 in]
              }
              frame "Busy" {
                n65 = call <vilib>:"Set Busy.vi"("error in (no error)"=w255) -> ("error out"=w254:errorcluster)  [unwired: 9 in, 1 out]
              }
            }
          }
          frame condition #1 {
          }
        }
        n66 = call <vilib>:"Add State(s) to Queue__JKI_lib_State_Machine.vi"("State(s) in (\"\")"=w248) -> ("States Out"=w247:string)  [unwired: 14 in]
      }
      frame "UI: Front Panel State" {
        # "Argument"
        n67 = Unbundle By Name(w260) -> ("Core.Current VI Reference"=w259:refnum<vi>)
        n68 = case shown="\"Hidden\", \"Hide\"" w258 {
          tunnel: w262 -> [w270 w285 w296 w309 w322]
          tunnel: [w272 w286 w298 w311 w324] -> w261
          tunnel: w259 -> [w271 w283 w297 w310 w323]
          frame "Open", "Standard", Default {
            w265 = T2."Standard" ("State")
            n69 = property class="VI"(reference=w271, error in=w270) -> (reference out=w268:refnum<vi>, error out=w269:errorcluster, "FP.State"=w267:T2)
            n70 = Not Equal?(x=w267, y=w265) -> (x != y?=w266:bool)
            n71 = case shown="True" w266 {
              tunnel: [w276 w278] -> w272
              tunnel: w269 -> [w275 w278]
              tunnel: w268 -> [w274 _]
              tunnel: w265 -> [w273 _]
              frame True {
                n72 = invoke class="VI" method="FP.Open"(reference=w274, error in=w275, "Activate"=TRUE, "State"=w273) -> (error out=w276:errorcluster)  [unwired: 1 in, 4 out]
              }
              frame False {
              }
            }
          }
          frame "Close", "Closed" {
            n73 = property class="VI"(reference=w283, error in=w285) -> (reference out=w282:refnum<vi>, error out=w284:errorcluster, "FP.State"=w280:T2)
            n74 = Not Equal?(x=w280, y=T2."Closed" ("Front Panel Window:State")) -> (x != y?=w279:bool)
            n75 = case shown="True" w279 {
              tunnel: [w287 w290] -> w286
              tunnel: w284 -> [w287 w289]
              tunnel: w282 -> [_ w288]
              frame False {
              }
              frame True {
                n76 = invoke class="VI" method="FP.Close"(reference=w288, error in=w289) -> (error out=w290:errorcluster)  [unwired: 1 in, 2 out]
              }
            }
          }
          frame "Hidden", "Hide" {
            w291 = T2."Hidden" ("State")
            n77 = property class="VI"(reference=w297, error in=w296) -> (reference out=w294:refnum<vi>, error out=w295:errorcluster, "FP.State"=w293:T2)
            n78 = Not Equal?(x=w293, y=w291) -> (x != y?=w292:bool)
            n79 = case shown="True" w292 {
              tunnel: [w302 w303] -> w298
              tunnel: w295 -> [w301 w303]
              tunnel: w294 -> [w300 _]
              tunnel: w291 -> [w299 _]
              frame True {
                n80 = invoke class="VI" method="FP.Open"(reference=w300, error in=w301, "State"=w299) -> (error out=w302:errorcluster)  [unwired: 2 in, 4 out]
              }
              frame False {
              }
            }
          }
          frame "Minimize", "Minimized" {
            w304 = T2."Minimized" ("State")
            n81 = property class="VI"(reference=w310, error in=w309) -> (reference out=w307:refnum<vi>, error out=w308:errorcluster, "FP.State"=w306:T2)
            n82 = Not Equal?(x=w306, y=w304) -> (x != y?=w305:bool)
            n83 = case shown="False" w305 {
              tunnel: [w315 w316] -> w311
              tunnel: w308 -> [w314 w316]
              tunnel: w307 -> [w313 _]
              tunnel: w304 -> [w312 _]
              frame True {
                n84 = invoke class="VI" method="FP.Open"(reference=w313, error in=w314, "State"=w312) -> (error out=w315:errorcluster)  [unwired: 2 in, 4 out]
              }
              frame False {
              }
            }
          }
          frame "Maximize", "Maximized" {
            w317 = T2."Maximized" ("State")
            n85 = property class="VI"(reference=w323, error in=w322) -> (reference out=w320:refnum<vi>, error out=w321:errorcluster, "FP.State"=w319:T2)
            n86 = Not Equal?(x=w319, y=w317) -> (x != y?=w318:bool)
            n87 = case shown="True" w318 {
              tunnel: [w328 w329] -> w324
              tunnel: w321 -> [w327 w329]
              tunnel: w320 -> [w326 _]
              tunnel: w317 -> [w325 _]
              frame True {
                n88 = invoke class="VI" method="FP.Open"(reference=w326, error in=w327, "State"=w325) -> (error out=w328:errorcluster)  [unwired: 2 in, 4 out]
              }
              frame False {
              }
            }
          }
        }
        n89 = call <vilib>:"Add State(s) to Queue__JKI_lib_State_Machine.vi"("State(s) in (\"\")"=w264) -> ("States Out"=w263:string)  [unwired: 14 in]
      }
      frame "---------- Macro ----------" {
        n90 = call <vilib>:"Add State(s) to Queue__JKI_lib_State_Machine.vi"("State(s) in (\"\")"=w334) -> ("States Out"=w333:string)  [unwired: 14 in]
      }
      frame "Macro: Initialize" {
        w336 = "Data: Initialize\nInitialize Core Data\nEvents: Register\nUI: Initialize\nUI: Front Panel State >> Open"  # Data: Initialize Initialize Core Data Events: Register UI: Initialize UI: Front Panel State >> Open
        n91 = call <vilib>:"Add State(s) to Queue__JKI_lib_State_Machine.vi"("State(s) in Front (\"\")"=w336, "State(s) in (\"\")"=w340) -> ("States Out"=w339:string)  [unwired: 13 in]
      }
      frame "Macro: Exit" {
        n92 = Unbundle By Name(w349) -> ("Core.Close Panel on Exit?"=w348:bool)
        n93 = Select(t="UI: Front Panel State >> Close", s=w348, f="") -> (s? t:f=w345:string)
        n94 = call <vilib>:"Add State(s) to Queue__JKI_lib_State_Machine.vi"("State(s) in Front (\"\")"="//Exit Sub-Modules ", "State(s) in (\"\")"=w345, "State(s) at Back (\"\")"="Data: Cleanup\nEvents: Unregister\nExit") -> ("States Out"=w343:string)  [unwired: 12 in]
        n95 = call <vilib>:"Add State(s) to Queue__JKI_lib_State_Machine.vi"("State(s) in Front (\"\")"=w343, "State(s) in (\"\")"=w352) -> ("States Out"=w351:string)  [unwired: 13 in]
      }
      frame "---------- API ----------" {
      }
      frame "API: API1" {
        n96 = call <userlib>:"CSM - Convert HexStr to Data.vi"("HEX String"=w357) -> ()  [unwired: 7 in, 2 out]
      }
      frame "API: API2" {
      }
      frame "asdfasd" {
      }
      frame "---------- Action ----------" {
        n97 = call <vilib>:"Add State(s) to Queue__JKI_lib_State_Machine.vi"("State(s) in Front (\"\")"="JUr‚ÑS\u0004\\¹pÑS" ("State(s) in Front (\"\")"), "State(s) in (\"\")"=w376) -> ("States Out"=w375:string)  [unwired: 13 in]
      }
      frame "Action: action1" {
        n98 = call <vilib>:"Add State(s) to Queue__JKI_lib_State_Machine.vi"("State(s) in (\"\")"=w381) -> ("States Out"=w380:string)  [unwired: 14 in]
      }
      frame "Action: action2" {
        n99 = call <vilib>:"Add State(s) to Queue__JKI_lib_State_Machine.vi"("State(s) in (\"\")"=w386) -> ("States Out"=w385:string)  [unwired: 14 in]
      }
    }
  }
  n100 = control-ref of="Current VI Reference"() -> (w24:refnum<vi>)
  n101 = call-poly "CSM-Helper API.vi"("VI"=w24) -> ("error out"=w22:errorcluster, "CSM-Helper.lvclass"=w23:refnum<class "CSM-Helper.lvclass">)  [unwired: 9 in]
  n102 = call "Read User-Defined States.vi"("error in (no error)"=w22, "CSM-Helper in"=w23) -> ("error out"=w14:errorcluster, "Array"=→"Array":string[], "CSM-Helper out"=w15:refnum<class "CSM-Helper.lvclass">)  [unwired: 7 in]
  n103 = call "Set Wire Label Visible.vi"("error in (no error)"=w14, "Connected Wire.Label.Visible"=FALSE, "CSM-Helper in"=w15) -> ("error out"=w17:errorcluster, "CSM-Helper out"=w18:refnum<class "CSM-Helper.lvclass">)  [unwired: 7 in]
  n104 = call "Read States.vi"("error in (no error)"=w17, "CSM-Helper in"=w18) -> ("error out"=w11:errorcluster, "Value"=w7:string[], "CSM-Helper out"=w10:refnum<class "CSM-Helper.lvclass">)  [unwired: 7 in]
  n105 = for {
    shift-right: [w391] -> w4
    shift-left: w11 -> [w394]
    shift-right: [w392] -> w5
    shift-left: w10 -> [w393]
    tunnel: w7 -> [w387] mode=indexing
    tunnel: [w388] -> w9 mode=indexing
    n106 = call "Get API Interface Info.vi"("error in (no error)"=w394, "CASE"=w387, "CSM-Helper in"=w393) -> ("error out"=w391:errorcluster, "Response"=w390:T1, "Argument"=w389:T1, "CSM-Helper out"=w392:refnum<class "CSM-Helper.lvclass">)  [unwired: 5 in]
    n107 = Bundle(w387, "Argument"=w389, "Response"=w390) -> (w388:cluster{string, "Argument":T1, "Response":T1})  [unwired: 1 in]
  }
  "Array 3" <- w9
  n108 = call "Get CaseFrame Reference By CaseName.vi"("error in (no error)"=w4, "CASE"="Data: Initialize", "CSM-Helper in"=w5) -> ("error out"=w3:errorcluster, "CSM-Helper out"=w2:refnum<class "CSM-Helper.lvclass">)  [unwired: 6 in, 1 out]
  n109 = call "Read States.vi"("error in (no error)"=w3, "CSM-Helper in"=w2) -> ("error out"=w12:errorcluster, "Value"=→"Array 2":string[], "CSM-Helper out"=w13:refnum<class "CSM-Helper.lvclass">)  [unwired: 7 in]
  n110 = call "Destroy.vi"("error in (no error)"=w12, "CSM-Helper in"=w13) -> ("error out"=w21:errorcluster)  [unwired: 8 in, 1 out]
  n111 = call <userlib>:"CSM - Send Message and Wait for Reply.vi"("Error In (no error)"=w21, "Target Module"="CSM", "State"="Macro: Exit") -> ()  [unwired: 6 in, 3 out]
